vi "Reset AI Tasks.vi"(8 "error in":errorcluster, 11 "cCRDS in":refnum<class "cCRDS.lvclass">=refnum) -> (0 "error out":errorcluster, 3 "cCRDS out":refnum<class "cCRDS.lvclass">)   [LabVIEW 2015, in "cCRDS.lvclass"]
uses:
  cCRDS.lvclass
  cCRDS.lvclass/cCRDS.ctl
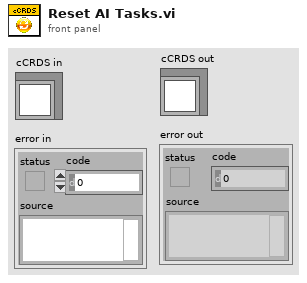
[diagram p1: front panel]
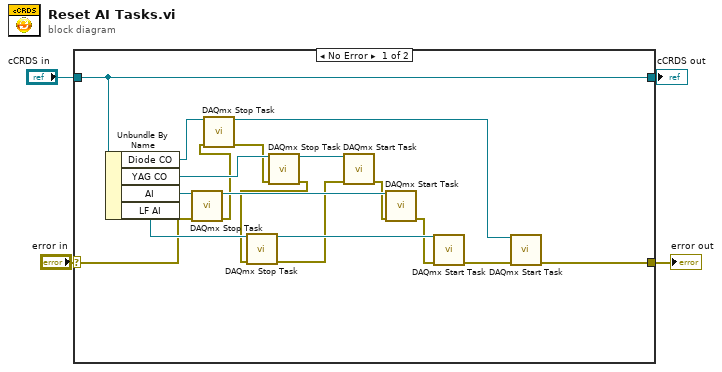
[diagram p0: block diagram]
diagram:
  n1 = case shown="No Error" "error in" {
    selector: "error in" -> [w17 w24]
    tunnel: [w10 w24] -> w3
    tunnel: [w22 w23] -> w1
    tunnel: "cCRDS in" -> [w22 w23]
    frame No Error {
      n2 = Unbundle By Name(w22) -> ("Diode CO"=w15:refnum<k21>, "YAG CO"=w14:refnum<k21>, "AI"=w16:refnum<k21>, "LF AI"=w21:refnum<k21>)
      n3 = call <vilib>:"DAQmx Stop Task.vi"("task/channels in"=w16, "error in"=w17) -> ("task out"=w20:refnum<k21>, "error out"=w9:errorcluster)  [unwired: 12 in]
      n4 = call <vilib>:"DAQmx Stop Task.vi"("task/channels in"=w15, "error in"=w9) -> ("task out"=w11:refnum<k21>, "error out"=w8:errorcluster)  [unwired: 12 in]
      n5 = call <vilib>:"DAQmx Stop Task.vi"("task/channels in"=w14, "error in"=w8) -> ("task out"=w13:refnum<k21>, "error out"=w7:errorcluster)  [unwired: 12 in]
      n6 = call <vilib>:"DAQmx Stop Task.vi"("task/channels in"=w21, "error in"=w7) -> ("task out"=w19:refnum<k21>, "error out"=w6:errorcluster)  [unwired: 12 in]
      n7 = call <vilib>:"DAQmx Start Task.vi"("task/channels in"=w13, "error in"=w6) -> ("error out"=w5:errorcluster)  [unwired: 12 in, 1 out]
      n8 = call <vilib>:"DAQmx Start Task.vi"("task/channels in"=w20, "error in"=w5) -> ("error out"=w18:errorcluster)  [unwired: 12 in, 1 out]
      n9 = call <vilib>:"DAQmx Start Task.vi"("task/channels in"=w19, "error in"=w18) -> ("error out"=w12:errorcluster)  [unwired: 12 in, 1 out]
      n10 = call <vilib>:"DAQmx Start Task.vi"("task/channels in"=w11, "error in"=w12) -> ("error out"=w10:errorcluster)  [unwired: 12 in, 1 out]
    }
    frame Error {
    }
  }
  "error out" <- w3
  "cCRDS out" <- w1
